vi "FlattenToXMLInternal.vi"(0 "Object in":refnum<class "OpenG_Object.lvclass">, 9 "require data consistency (T)":bool=TRUE, 11 "error in (no error)":errorcluster, 12 "timeout in ms (-1)":i32=-1) -> (4 "Object out":refnum<class "OpenG_Object.lvclass">, 6 "Object as XML":string="\n", 8 "Before Child":string, 10 "After Child":string="\n", 14 "time left":i32=-1, 15 "error out":errorcluster)   [LabVIEW 2020, in "OpenG_Object.lvclass"]
doc: "Internal method to flatten object content to XML."
uses:
  OpenG_Object.lvclass
  OpenG_Object.lvclass/OpenG_Object.ctl
panel:
  # "Please visit http://www.OpenG.org to learn about the\nOpen Source LabVIEW software movement.\n\nNOTICE -- YOU MUST LEAVE THIS NOTICE IN PLACE.  PER THE TERMS OF THE LICENSE BELOW, YOU MAY SUBLICENSE THIS SOFTWARE \nIN ANY WAY THAT DOES NOT CONFLICT WITH THIS LICENSE.\n\n### BSD License (http://www.opensource.org/licenses/bsd-license.php) Begin ###\n\nCopyright (c) 2007, Tomi Maila\nCopyright (c) 2007, Endevo AB\n\n\nAll rights reserved.\n\nRedistribution and use in source and binary forms, with or without modification, are permitted provided that the following conditions are met:\n\n    * Redistributions of source code must retain the above copyright notice, this list of conditions and the following disclaimer.\n    * Redistributions in binary form must reproduce the above copyright notice, this list of conditions and the following disclaimer in the \n       documentation and/or other materials provided with the distribution.\n    * Neither the name of Endevo AB nor the names of the contributors may be used to endorse or promote products derived\n       from this software without specific prior written permission.\n\nTHIS SOFTWARE IS PROVIDED BY THE COPYRIGHT HOLDERS AND CONTRIBUTORS \"AS IS\" AND ANY EXPRESS OR IMPLIED WARRANTIES, \nINCLUDING, BUT NOT LIMITED TO, THE IMPLIED WARRANTIES OF MERCHANTABILITY AND FITNESS FOR A PARTICULAR PURPOSE ARE \nDISCLAIMED. IN NO EVENT SHALL THE COPYRIGHT OWNER OR CONTRIBUTORS BE LIABLE FOR ANY DIRECT, INDIRECT, INCIDENTAL,\n SPECIAL, EXEMPLARY, OR CONSEQUENTIAL DAMAGES (INCLUDING, BUT NOT LIMITED TO, PROCUREMENT OF SUBSTITUTE GOODS OR \nSERVICES; LOSS OF USE, DATA, OR PROFITS; OR BUSINESS INTERRUPTION) HOWEVER CAUSED AND ON ANY THEORY OF LIABILITY, \nWHETHER IN CONTRACT, STRICT LIABILITY, OR TORT (INCLUDING NEGLIGENCE OR OTHERWISE) ARISING IN ANY WAY OUT OF THE USE \nOF THIS SOFTWARE, EVEN IF ADVISED OF THE POSSIBILITY OF SUCH DAMAGE.\n\n### BSD License End ###"
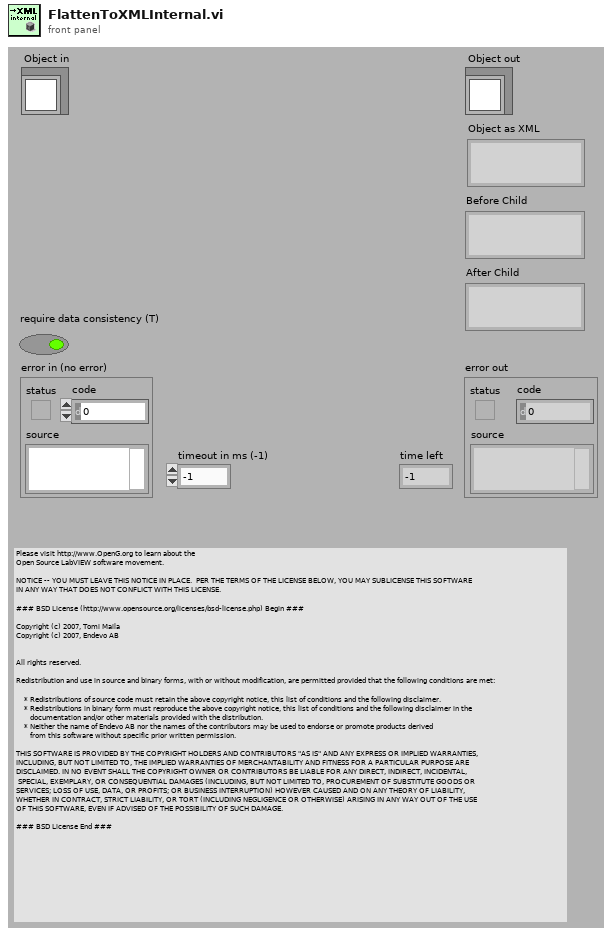
[diagram p1: front panel]
types:
  T1 = cluster{"Major":u16, "Minor":u16, "Fix":u16, "Build":u16}
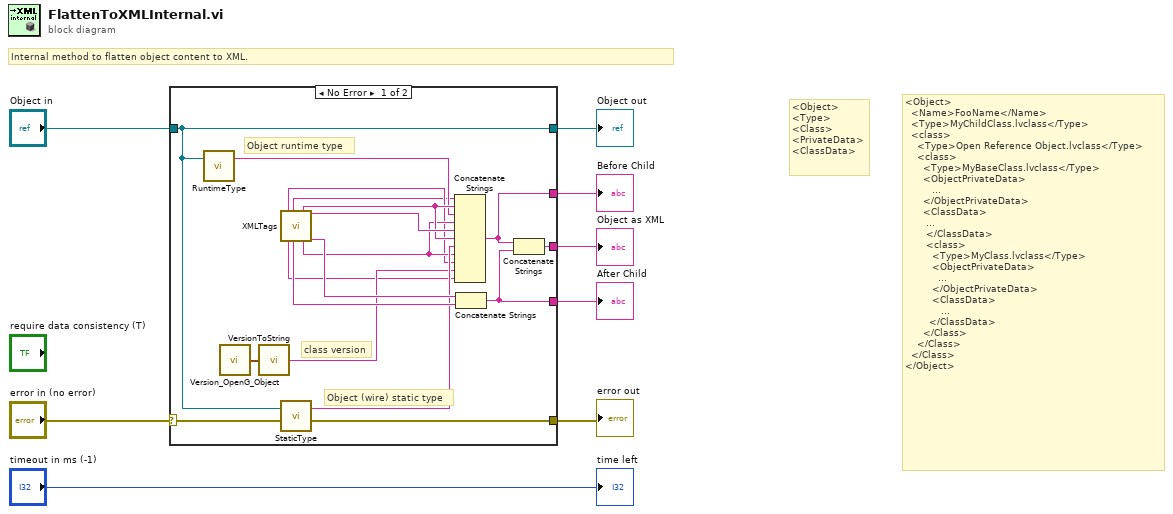
[diagram p0: block diagram]
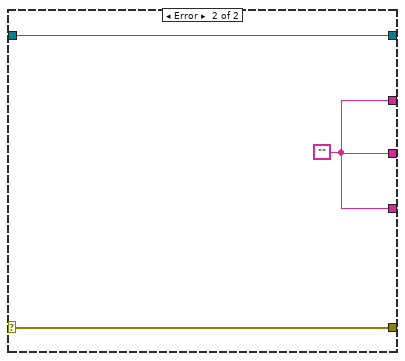
[diagram p2: hidden frame]
diagram:
  # "Internal method to flatten object content to XML."
  # "<Object>\n<Type>\n<Class>\n<PrivateData>\n<ClassData>"
  # "<Object>\n  <Name>FooName</Name>\n  <Type>MyChildClass.lvclass</Type>\n  <class>\n    <Type>Open Reference Object.lvclass</Type>\n    <class>\n      <Type>MyBaseClass.lvclass</Type>\n\t     <ObjectPrivateData>\n\t        ...\n\t     </ObjectPrivateData>\n\t     <ClassData>\n\t      ...\n\t      </ClassData>\n\t      <class>\n\t        <Type>MyClass.lvclass</Type>\n\t        <ObjectPrivateData>\n\t          ...\n\t        </ObjectPrivateData>\n\t        <ClassData>\n\t           ...\n\t       </ClassData>\n      </Class>\n    </Class>\n  </Class>\n</Object>"
  n1 = case shown="No Error" "error in (no error)" {
    selector: "error in (no error)" -> [w22 w27]
    tunnel: "Object in" -> [w10 w29]
    tunnel: [w26 w27] -> w7
    tunnel: [w25 w28] -> w6
    tunnel: [w24 w28] -> w5
    tunnel: [w23 w28] -> w4
    tunnel: [w10 w29] -> w3
    frame No Error {
      # "class version"
      # "Object (wire) static type"
      # "Object runtime type"
      n2 = call "RuntimeType.vi"("Object in"=w10) -> ("runtime class name"=w12:string)  [unwired: 2 in]
      n3 = call "Version_OpenG_Object.vi"() -> ("Version"=w11:T1)
      n4 = call "VersionToString.vi"("Version"=w11) -> ("Version as string"=w14:string)
      n5 = call "XMLTags.vi"() -> ("<Version>"=w15:string, "</Version>"=w13:string, "<Object>"=w9:string, "</Object>"=w19:string, "<Type>"=w18:string, "</Type>"=w16:string, "<Class>"=w21:string, "</Class>"=w20:string)  [unwired: 4 in, 8 out]
      n6 = call "StaticType.vi"("error in (no error)"=w22, "Object in"=w10) -> ("error out"=w26:errorcluster, "static class name"=w17:string)  [unwired: 5 in]
      n7 = Concatenate Strings(w9, w18, w12, w16, w21, w18, w17, w16, w15, w14, w13) -> (w24:string)
      n8 = Concatenate Strings(w20, w19) -> (w23:string)
      n9 = Concatenate Strings(w24, w23) -> (w25:string)
    }
    frame Error {
      w28 = ""
    }
  }
  "error out" <- w7
  "Object out" <- w3
  "Object as XML" <- w6
  "Before Child" <- w5
  "After Child" <- w4
  "time left" <- "timeout in ms (-1)"
